vi "Display.vi"(6 "Text to Display(empty)":string, 7 "Set/Check (F:Set)":bool, 8 "error in (no error)":errorcluster, 9 "Clear Display (F:No)":bool, 10 "Instrument Display (T:On)":bool=TRUE, 11 "VISA Resource Name":refnum<visa-resource-name>) -> (0 "error out":errorcluster, 1 "Display Enabled":bool, 2 "Displayed Text?":string, 3 "VISA Resource Name Out":refnum<visa-resource-name>)   [LabVIEW 2012, in "Agilent 34970.lvlib"]
doc: "This VI allows you to set or check the instrument's display. You can clear, turn on/off, or display a text message. You can also determine what is currently being displayed, or if the display is on/off."
uses:
  <instrlib>/Agilent 34970/Agilent 34970.lvlib
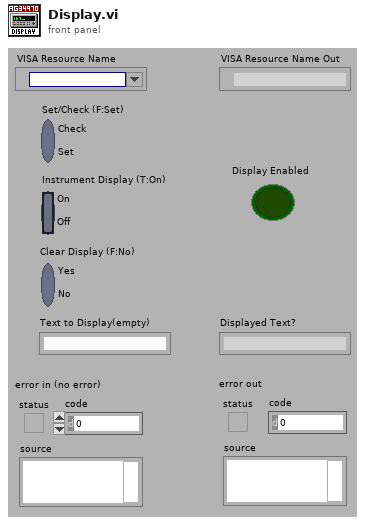
[diagram p1: front panel]
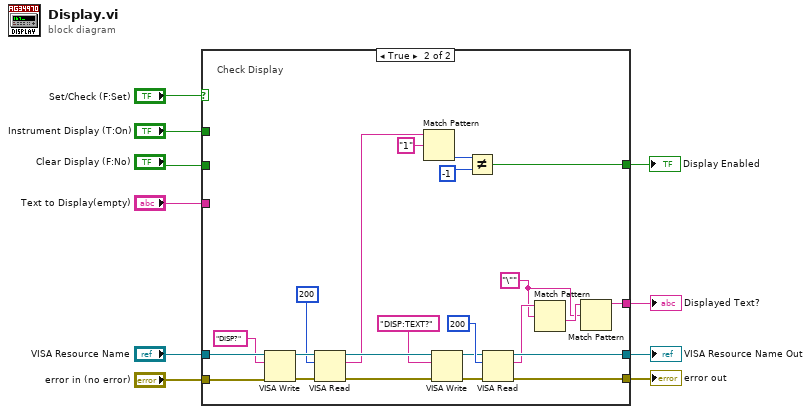
[diagram p0: block diagram]
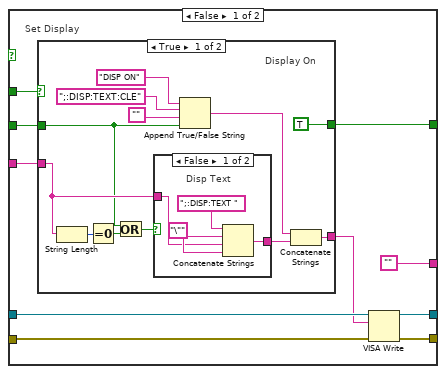
[diagram p2: hidden frame]
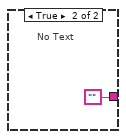
[diagram p3: hidden frame]
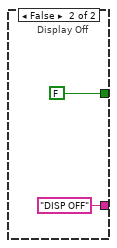
[diagram p4: hidden frame]
diagram:
  n1 = case shown="True" "Set/Check (F:Set)" {
    tunnel: "Clear Display (F:No)" -> [w11 _]
    tunnel: "Instrument Display (T:On)" -> [w12 _]
    tunnel: "Text to Display(empty)" -> [w20 _]
    tunnel: "VISA Resource Name" -> [w19 w62]
    tunnel: [w16 w53] -> w4
    tunnel: [w17 w52] -> w3
    tunnel: "error in (no error)" -> [w18 w51]
    tunnel: [w14 w44] -> w2
    tunnel: ["" w40] -> w1
    frame False {
      # "Set Display"
      n2 = case shown="True" w12 {
        tunnel: w20 -> [w31 _]
        tunnel: [TRUE FALSE] -> w14
        tunnel: [w28 "DISP OFF"] -> w15
        tunnel: w11 -> [w21 _]
        frame True {
          # "Display On"
          n3 = String Length(string=w31) -> (length=w32:i32)
          n4 = Equal To 0?(x=w32) -> (x = 0?=w30:bool)
          n5 = Or(x=w21, y=w30) -> (x .or. y?=w29:bool)
          n6 = case shown="False" w29 {
            tunnel: w31 -> [w35 _]
            tunnel: [w33 ""] -> w27
            frame False {
              w36 = "\""
              # "Disp Text"
              n7 = Concatenate Strings(";:DISP:TEXT ", w36, w35, w36) -> (w33:string)
            }
            frame True {
              # "No Text"
            }
          }
          n8 = Append True/False String(1:w21, 2:"", 3:";:DISP:TEXT:CLE" ("true string"), 4:"DISP ON" ("string (\"\")")) -> (0:w26:string)
          n9 = Concatenate Strings(w26, w27) -> (w28:string)
        }
        frame False {
          # "Display Off"
        }
      }
      n10 = VISA Write(VISA resource name=w19, write buffer=w15, error in (no error)=w18) -> (VISA resource name out=w16:refnum<visa-resource-name>, error out=w17:errorcluster)  [unwired: 1 out]
    }
    frame True {
      w41 = "\"" ("regular expression")
      # "Check Display"
      n11 = VISA Write(VISA resource name=w62, write buffer="DISP?", error in (no error)=w51) -> (VISA resource name out=w61:refnum<visa-resource-name>, error out=w60:errorcluster)  [unwired: 1 out]
      n12 = VISA Read(VISA resource name=w61, byte count=u32 200 ("byte count (0)"), error in (no error)=w60) -> (VISA resource name out=w56:refnum<visa-resource-name>, read buffer=w48:string, error out=w55:errorcluster)  [unwired: 1 out]
      n13 = Match Pattern(string=w48, regular expression="1") -> (offset past match=w46:i32)  [unwired: 1 in, 3 out]
      n14 = VISA Write(VISA resource name=w56, write buffer="DISP:TEXT?", error in (no error)=w55) -> (VISA resource name out=w57:refnum<visa-resource-name>, error out=w54:errorcluster)  [unwired: 1 out]
      n15 = Not Equal?(x=w46, y=-1) -> (x != y?=w44:bool)
      n16 = VISA Read(VISA resource name=w57, byte count=u32 200 ("byte count (0)"), error in (no error)=w54) -> (VISA resource name out=w53:refnum<visa-resource-name>, read buffer=w42:string, error out=w52:errorcluster)  [unwired: 1 out]
      n17 = Match Pattern(string=w42, regular expression=w41) -> (after substring=w43:string)  [unwired: 1 in, 3 out]
      n18 = Match Pattern(string=w43, regular expression=w41) -> (before substring=w40:string)  [unwired: 1 in, 3 out]
    }
  }
  "Displayed Text?" <- w1
  "VISA Resource Name Out" <- w4
  "error out" <- w3
  "Display Enabled" <- w2
